vi "Build path.vi"(5 "Required?":bool, 7 "String":string, 10 "error in":errorcluster, 11 "Path":path) -> (2 "error out":errorcluster, 3 "Path Out":path)   [LabVIEW 2023, in "Report.lvlib" / "Report.lvclass"]
uses:
  Report.lvclass
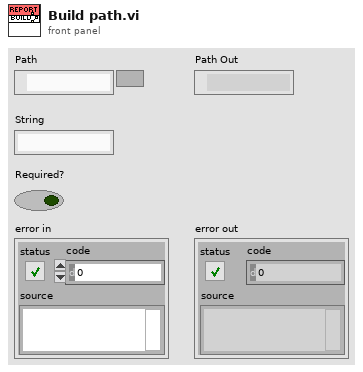
[diagram p1: front panel]
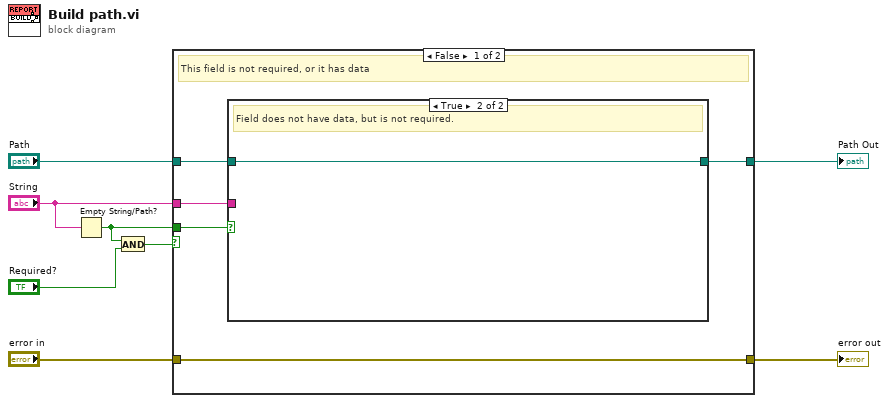
[diagram p0: block diagram]
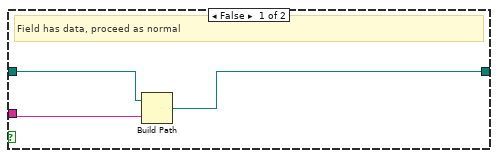
[diagram p2: hidden frame]
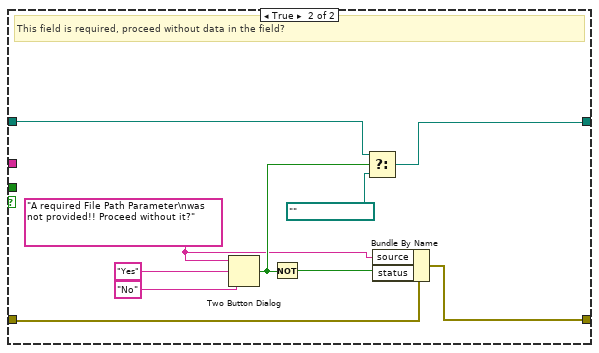
[diagram p3: hidden frame]
diagram:
  n1 = Empty String/Path?(string/path="String") -> (empty?=w2:bool)
  n2 = And(x=w2, y="Required?") -> (x .and. y?=w8:bool)
  n3 = case shown="False" w8 {
    tunnel: "error in" -> [w13 w21]
    tunnel: "Path" -> [w11 w24]
    tunnel: [w10 w22] -> w5
    tunnel: [w13 w18] -> w4
    tunnel: w2 -> [w12 _]
    tunnel: "String" -> [w9 _]
    frame False {
      # "This field is not required, or it has data"
      n4 = case shown="True" w12 {
        tunnel: w11 -> [w16 w17]
        tunnel: [w14 w17] -> w10
        tunnel: w9 -> [w15 _]
        frame False {
          # "Field has data, proceed as normal"
          n5 = Build Path(base path=w16, name or relative path=w15) -> (appended path=w14:path)
        }
        frame True {
          # "Field does not have data, but is not required."
        }
      }
    }
    frame True {
      w19 = "A required File Path Parameter\nwas not provided!! Proceed without it?" ("message")
      # "This field is required, proceed without data in the field?"
      n6 = Two Button Dialog(message=w19, 1:"No" ("F button name (\"Cancel\")"), 2:"Yes" ("T button name (\"OK\")")) -> (T button?=w25:bool)
      n7 = Not(x=w25) -> (.not. x?=w20:bool)
      n8 = Select(t=w24, s=w25, f=path "") -> (s? t:f=w22:path)
      n9 = Bundle By Name(cluster=w21, "source"=w19, "status"=w20) -> (w18:errorcluster)
    }
  }
  "error out" <- w4
  "Path Out" <- w5
